vi "average data.vi"(8 "error in (no error)":errorcluster, 9 "setpoints":T2={"target clarified turbidity (NTU)"=0.3, "flocculator volume (L)"=0.0, "clarifier volume (L)"=0.0, "dose updates per HRT"=1} {"target clarified turbidity (NTU)" min=0.1 max=5.0 step=0.01; "dose updates per HRT" min=1 max=1000 step=1}, 10 "data input":T3, 11 "seconds since 1Jan1904":timestamp) -> (0 "error out":errorcluster, 1 "new interval":bool, 3 "averaged data":T1)   [LabVIEW 2019]
uses:
  setpoints.ctl
  data cluster.ctl
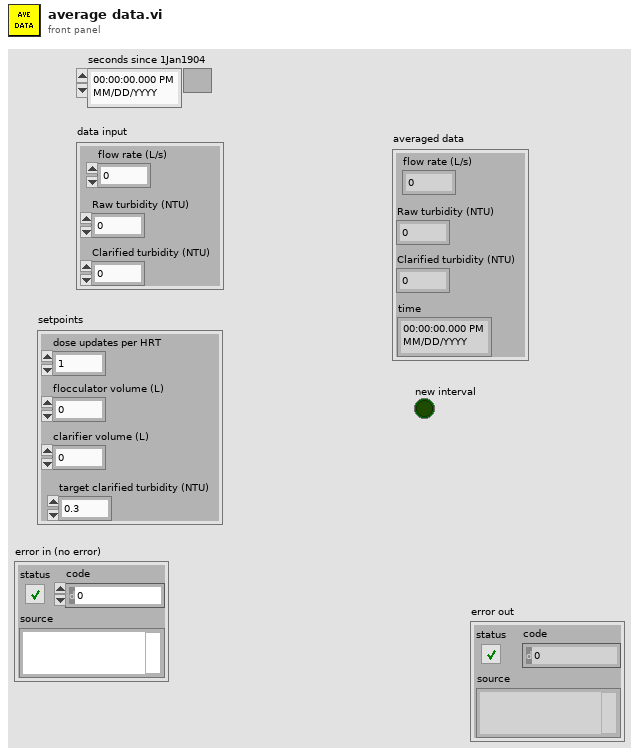
[diagram p1: front panel]
types:
  T1 = typedef "data cluster.ctl" = cluster{"Clarified turbidity (NTU)":dbl, "Raw turbidity (NTU)":dbl, "flow rate (L/s)":dbl, "time":timestamp}
  T2 = typedef "setpoints.ctl" = cluster{"target clarified turbidity (NTU)":dbl, "flocculator volume (L)":dbl, "clarifier volume (L)":dbl, "dose updates per HRT":u32}
  T3 = cluster{"Clarified turbidity (NTU)":dbl, "Raw turbidity (NTU)":dbl, "flow rate (L/s)":dbl}
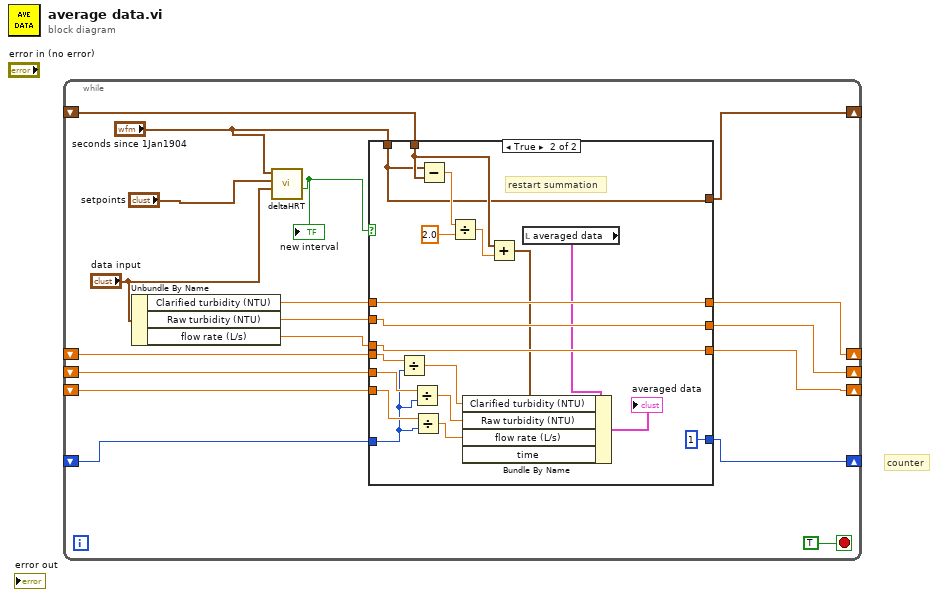
[diagram p0: block diagram]
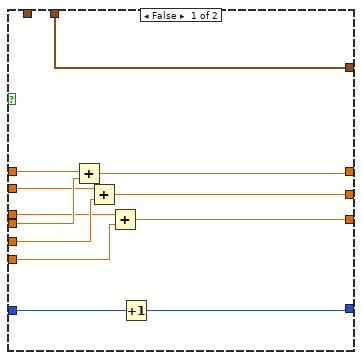
[diagram p2: hidden frame]
diagram:
  # "counter"
  n1 = while {
    shift-right: [w15] -> _
    shift-left: _ -> [w14]
    shift-right: [w17] -> _
    shift-left: _ -> [w16]
    shift-right: [w13] -> _
    shift-left: _ -> [w11]
    shift-right: [w9] -> _
    shift-left: _ -> [w8]
    shift-right: [w5] -> _
    shift-left: _ -> [w6]
    stop <- TRUE stop-if-true
    n2 = Unbundle By Name("data input") -> ("Clarified turbidity (NTU)"=w12:dbl, "Raw turbidity (NTU)"=w10:dbl, "flow rate (L/s)"=w7:dbl)
    n3 = call "deltaHRT.vi"("data input"="data input", "setpoints"="setpoints", "seconds since 1Jan1904"="seconds since 1Jan1904") -> ("new interval"=w3:bool)  [unwired: 6 in, 2 out]
    "new interval" <- w3
    n4 = case shown="True" w3 {
      tunnel: [w29 1] -> w17
      tunnel: w16 -> [w30 w39]
      tunnel: [w28 w31] -> w15
      tunnel: "seconds since 1Jan1904" -> [_ w31]
      tunnel: w14 -> [w28 w32]
      tunnel: [w25 w48] -> w13
      tunnel: w12 -> [w26 w48]
      tunnel: w11 -> [w27 w45]
      tunnel: w10 -> [w24 w47]
      tunnel: [w22 w47] -> w9
      tunnel: w8 -> [w23 w42]
      tunnel: w7 -> [w21 w46]
      tunnel: w6 -> [w20 w40]
      tunnel: [w19 w46] -> w5
      frame False {
        n5 = Add(x=w26, y=w27) -> (x+y=w25:dbl)
        n6 = Add(x=w24, y=w23) -> (x+y=w22:dbl)
        n7 = Add(x=w21, y=w20) -> (x+y=w19:dbl)
        n8 = Increment(x=w30) -> (x+1=w29:i32)
      }
      frame True {
        # "restart summation"
        n9 = Divide(x=w45, y=w39) -> (x/y=w43:dbl)
        n10 = Divide(x=w42, y=w39) -> (x/y=w41:dbl)
        n11 = Divide(x=w40, y=w39) -> (x/y=w38:dbl)
        n12 = Subtract(x=w31, y=w32) -> (x-y=w35:dbl)
        n13 = Divide(x=w35, y=2.0) -> (x/y=w34:dbl)
        n14 = Add(x=w32, y=w34) -> (x+y=w33:timestamp)
        n15 = local read "averaged data"() -> (w37:T1)
        n16 = Bundle By Name(cluster=w37, "Clarified turbidity (NTU)"=w43, "Raw turbidity (NTU)"=w41, "flow rate (L/s)"=w38, "time"=w33) -> (→"averaged data":T1)
      }
    }
  }
